vi "SV Read Data at Timestamp.vi"(6 "timestamp (first available)":timestamp format="%<%H:%M:%S%6u\n%x>T", 7 "reader ID":string="SubsetData", 8 "error in (no error)":errorcluster, 9 "timeout (0 ms)":i32, 10 "block length (-1 = all)":i32=-1, 11 "buffer":refnum<data-value>) -> (0 "error out":errorcluster, 1 "end of buffer":bool, 2 "waveforms subset":waveform(dbl)[](array[waveform]), 3 "buffer out":refnum<data-value>)   [LabVIEW 2017]
doc: "Adds buffering to stimulus-response applications. You must manually select the polymorphic instance to use."
uses:
  <vilib>/addons/_NISVFA/_Shared subVIs/Data Objects/Waveforms (DBL)/Waveforms (N Ch).lvclass
  C:/Program Files (x86)/National Instruments/LabVIEW 2017/vi.lib/addons/_NISVFA/_Shared subVIs/Data Objects/Data/Data.lvclass
  <vilib>/addons/_NISVFA/_Shared subVIs/Data Objects/Data/Data.lvclass/Data.ctl
  <vilib>/addons/_NISVFA/_Shared subVIs/Data Objects/Waveforms (DBL)/Waveforms (N Ch).lvclass/Waveforms (N Ch).ctl
  <vilib>/addons/_NISVFA/_Shared subVIs/Data Objects/Waveforms (DBL)/Read Mode for Deleting Stale Data.vi
  <vilib>/addons/_NISVFA/_Shared subVIs/Data Objects/subVIs/Get Data Timestamp.vi
  <vilib>/addons/_NISVFA/_Shared subVIs/Common/sv_Convert Timestamp to Relative Index.vi
  <vilib>/addons/_NISVFA/_Shared subVIs/Data Objects/subVIs/Get Data Length.vi
  <vilib>/addons/_NISVFA/_Shared subVIs/Common/SV Get Data Subset.vi
  <vilib>/addons/_NISVFA/_Shared subVIs/Common/svc_Copy Waveform Subset (Index).vi
  <vilib>/addons/_NISVFA/_Shared subVIs/Common/sv_Get NI Property Name String.vi
  <vilib>/addons/_NISVFA/_Shared subVIs/Data Objects/subVIs/Get Oldest of ReaderTimestamps.vi
  <vilib>/addons/_NISVFA/_Shared subVIs/Data Objects/subVIs/Set Data Timestamp.vi
  <vilib>/addons/_NISVFA/_Shared subVIs/Data Objects/subVIs/Set Data Length.vi
  <vilib>/addons/_NISVFA/_Shared subVIs/Common/svc_Get Waveform Subset (Index).vi
  <vilib>/addons/_NISVFA/_Shared subVIs/Common/svc_Copy Array Subset (Index).vi
  <vilib>/addons/_NISVFA/_Shared subVIs/Common/svc_Get Array Subset (Index).vi
  <vilib>/addons/_NISVFA/_Shared subVIs/Common/svc_Coerce Index and Length.vi
  <vilib>/addons/_NISVFA/_Shared subVIs/Common/svc_Conditional Merge Error.vi
  <vilib>/Utility/error.llb/Trim Whitespace.vi
  <vilib>/addons/_NISVFA/_Shared subVIs/Data Objects/Data/Data.lvclass
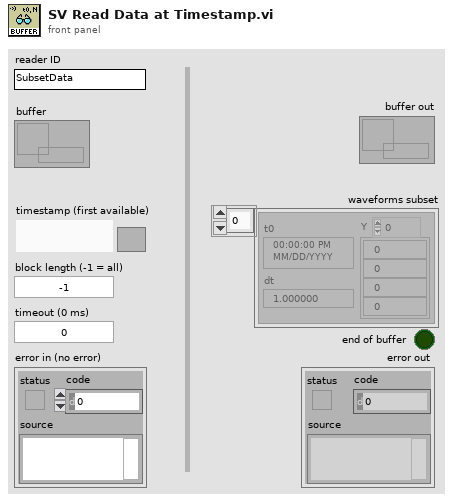
[diagram p1: front panel]
types:
  T1 = enum16{"Data Ready", "First Sample Not Yet Available", "Last Sample Not Yet Available", "Data No Longer Available"}
  T2 = typedef "svc_Delete Data Options (enum).ctl" = enum16{"Write", "Read", "Release"}
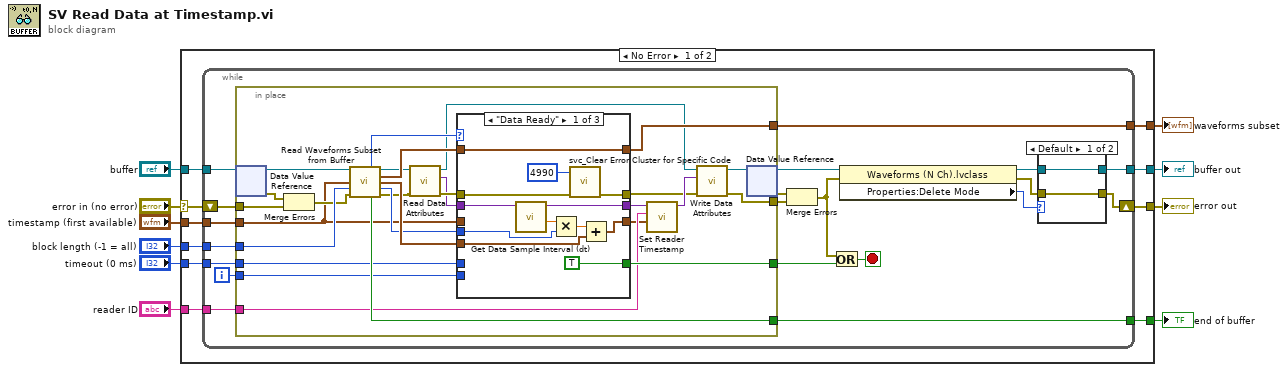
[diagram p0: block diagram]
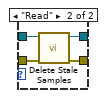
[diagram p2: hidden frame]
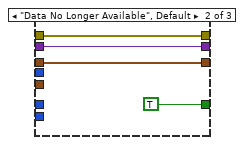
[diagram p3: hidden frame]
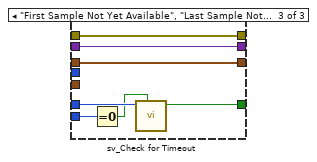
[diagram p4: hidden frame]
diagram:
  n1 = case shown="No Error" "error in (no error)" {
    selector: "error in (no error)" -> [w15 w97]
    tunnel: "buffer" -> [w14 w98]
    tunnel: "reader ID" -> [w20 _]
    tunnel: "timestamp (first available)" -> [w19 _]
    tunnel: [w13 w98] -> w7
    tunnel: [w12 w97] -> w6
    tunnel: "block length (-1 = all)" -> [w18 _]
    tunnel: [w17 _] -> w4
    tunnel: [w16 _] -> w3
    tunnel: "timeout (0 ms)" -> [w11 _]
    frame No Error {
      n2 = while {
        tunnel: w20 -> [w40]
        tunnel: w19 -> [w39]
        tunnel: w18 -> [w38]
        tunnel: [w37] -> w17
        tunnel: [w36] -> w16
        tunnel: w14 -> [w34]
        tunnel: [w25] -> w13
        shift-right: [w24] -> w12
        shift-left: w15 -> [w35]
        tunnel: w11 -> [w30]
        i -> [w31]
        stop <- w22 stop-if-true
        n3 = in-place {
          in-place-border: w40 -> [w55]
          in-place-border: w39 -> [w47]
          in-place-border: [w56] -> w32
          in-place-border: w38 -> [w73]
          in-place-border: [w68] -> w37
          in-place-border: [w67] -> w36
          in-place-border: w35 -> [w65]
          in-place-border: [w62] -> w21
          in-place-border: w31 -> [w61]
          in-place-border: w30 -> [w60]
          n4 = in-place-dvr #1(w34) -> (w66:refnum<class "Waveforms (N Ch).lvclass">, w63:errorcluster)
          n5 = Merge Errors(w63, w65) -> (w64:errorcluster)
          n6 = call <vilib>:"Read Waveforms Subset from Buffer.vi"("Waveforms (N Ch)"=w66, "timestamp"=w47, "block length"=w73, "error in (no error)"=w64) -> ("subset status"=w70:T1, "Waveforms (N Ch)"=w53:refnum<class "Waveforms (N Ch).lvclass">, "waveforms subset"=w69:waveform(dbl)[], "actual timestamp"=w72:timestamp, "actual length"=w71:i32, "end of buffer"=w67:bool, "error out"=w52:errorcluster)  [unwired: 5 in]
          n7 = call <vilib>:"Read Data Attributes.vi"("error in (no error)"=w52, "Data in"=w53) -> ("error out"=w51:errorcluster, "data attributes"=w49:variant, "Data out"=w50:refnum<class "Waveforms (N Ch).lvclass">)  [unwired: 7 in]
          n8 = case shown="\"Data Ready\"" w70 {
            tunnel: w51 -> [w78 w89 w93]
            tunnel: [w75 w89 w93] -> w57
            tunnel: w72 -> [w84 _ _]
            tunnel: w71 -> [w83 _ _]
            tunnel: w69 -> [w81 _ _]
            tunnel: [w81 _ _] -> w68
            tunnel: [TRUE TRUE w95] -> w62
            tunnel: w61 -> [_ _ w96]
            tunnel: w60 -> [_ _ w94]
            tunnel: [w77 w87 w91] -> w54
            tunnel: w49 -> [w76 w87 w91]
            tunnel: [w74 w86 w90] -> w48
            tunnel: w47 -> [_ w86 w90]
            frame "Data Ready" {
              n9 = call <vilib>:"Get Data Sample Interval (dt).vi"("variant in"=w76) -> ("dt [s]"=w82:dbl, "variant out"=w77:variant)  [unwired: 9 in]
              n10 = Multiply(x=w82, y=w83) -> (x*y=w85:dbl)
              n11 = call <vilib>:"svc_Clear Error Cluster for Specific Code.vi"("error in (no error)"=w78, "code"=4990) -> ("error out"=w75:errorcluster)  [unwired: 12 in, 1 out]
              n12 = Add(x=w85, y=w84) -> (x+y=w74:timestamp)
            }
            frame "Data No Longer Available", Default {
            }
            frame "First Sample Not Yet Available", "Last Sample Not Yet Available" {
              n13 = Equal To 0?(x=w96) -> (x = 0?=w92:bool)
              n14 = call <vilib>:"sv_Check for Timeout.vi"("reset"=w92, "timeout [ms]"=w94) -> ("timeout"=w95:bool)  [unwired: 8 in, 1 out]
            }
          }
          n15 = call <vilib>:"Set Reader Timestamp.vi"("timestamp"=w48, "ID"=w55, "data attributes in"=w54) -> ("data attributes out"=w59:variant)  [unwired: 8 in]
          n16 = call <vilib>:"Write Data Attributes.vi"("error in (no error)"=w57, "data attributes"=w59, "Data in"=w50) -> ("error out"=w56:errorcluster, "Data out"=w58:refnum<class "Waveforms (N Ch).lvclass">)  [unwired: 7 in]
          n17 = in-place-dvr #1(w58) -> (w26:refnum<data-value>, w33:errorcluster)
        }
        n18 = Merge Errors(w33, w32) -> (w23:errorcluster)
        n19 = Or(x=w23, y=w21) -> (x .or. y?=w22:bool)
        n20 = property class="Waveforms (N Ch).lvclass"(reference=w26, error in=w23) -> (reference out=w28:refnum<data-value>, error out=w27:errorcluster, "Properties:Delete Mode"=w29:T2)
        n21 = case shown="Default" w29 {
          tunnel: [w42 w45] -> w25
          tunnel: w28 -> [w42 w46]
          tunnel: w27 -> [w41 w44]
          tunnel: [w41 w43] -> w24
          frame Default {
          }
          frame "Read" {
            n22 = call <vilib>:"Delete Stale Samples.vi"("error in (no error)"=w44, "buffer"=w46) -> ("error out"=w43:errorcluster, "buffer"=w45:refnum<data-value>)  [unwired: 6 in, 2 out]
          }
        }
      }
    }
    frame Error {
    }
  }
  "buffer out" <- w7
  "error out" <- w6
  "waveforms subset" <- w4
  "end of buffer" <- w3
